vi "Write waveform to file.vi"(7 "File IO parameters":T1={"Output Folder"=path "C:/Users/Abigail/Documents/Imperial Optical software/Optical Software Code Simplified/Output", "Error file"=path "Error Log.txt", "Config file"=path "Config.ini", "File prefix"="", "Waveform read"={"t0"=timestamp(0 s since 1904-01-01), "dt"=1.0, "Y"=[]}}, 8 "error in":errorcluster, 10 "Dataset name":string="DAQ (raw data)", 11 "Data":dbl[][](array[numeric])) -> (0 "error out":errorcluster)   [LabVIEW 2017, in "File IO.lvlib"]
uses:
  File IO.lvlib
  Controls/Params.ctl
  <vilib>/Utility/file.llb/Write To Spreadsheet File (DBL).vi
panel:
  in  "Waveform":waveform(dbl)={"t0"=timestamp(3604668038.5453954 s since 1904-01-01), "dt"=1.0, "Y"=array[495 elements]}
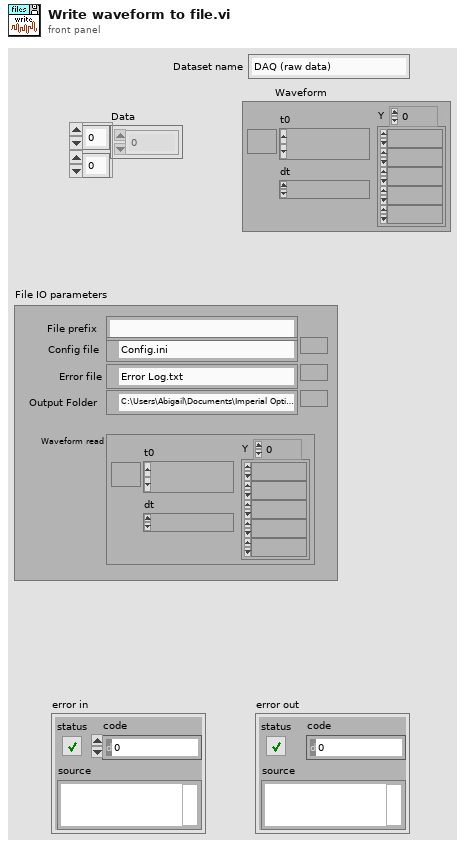
[diagram p1: front panel]
types:
  T1 = typedef "File IO.lvlib/Params.ctl" = cluster{"Output Folder":path, "Error file":path, "Config file":path, "File prefix":string, "Waveform read":waveform(dbl)}
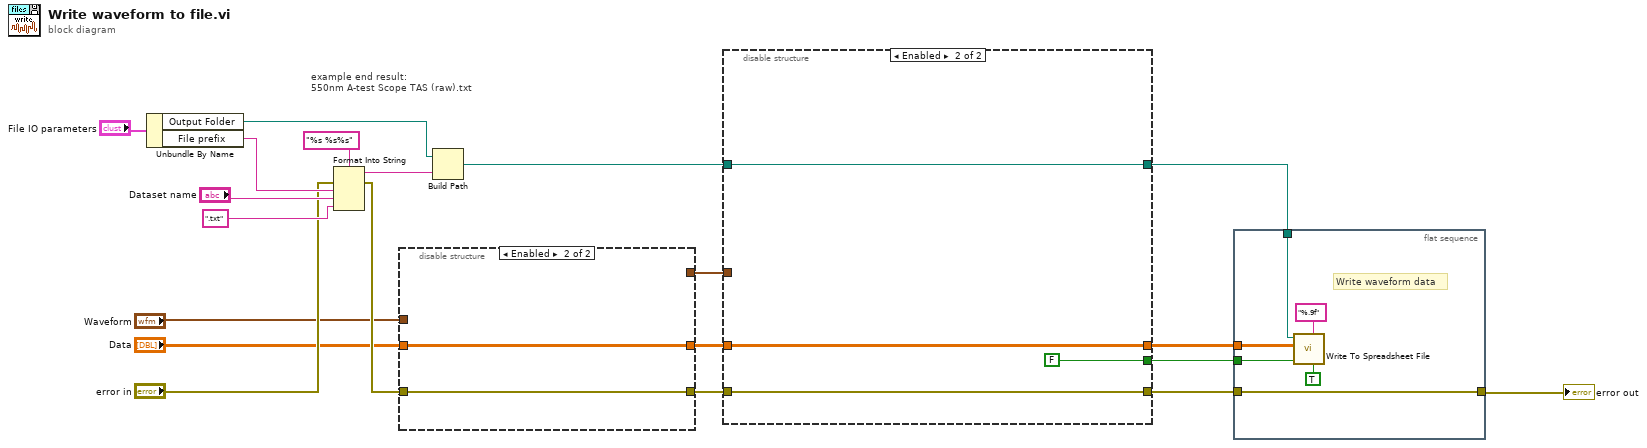
[diagram p0: block diagram]
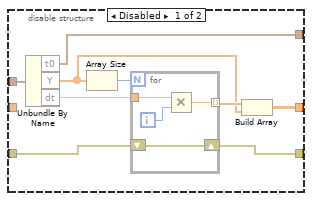
[diagram p2: hidden frame]
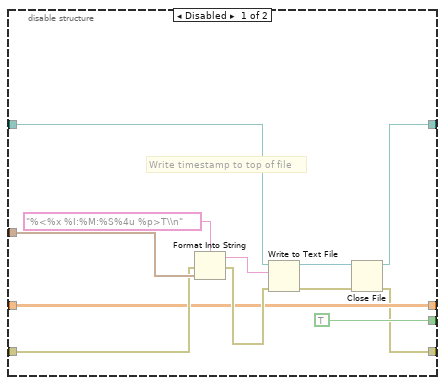
[diagram p3: hidden frame]
diagram:
  # "example end result:\n550nm A-test Scope TAS (raw).txt"
  n1 = Unbundle By Name("File IO parameters") -> ("Output Folder"=w20:path, "File prefix"=w19:string)
  n2 = Format Into String(format string="%s %s%s", error in="error in", w19, "Dataset name", ".txt" ("Dataset name 2")) -> (resulting string=w15:string, error out=w12:errorcluster)  [unwired: 1 in]
  n3 = disable-structure shown="Enabled" {
    disable-tunnel: w12 -> [w27 w34]
    disable-tunnel: "Waveform" -> [w24 _]
    disable-tunnel: [w23 _] -> w9
    disable-tunnel: [w22 w34] -> w8
    disable-tunnel: [w21 w35] -> w4
    disable-tunnel: "Data" -> [_ w35]
    frame Disabled {
      n4 = Unbundle By Name(w24) -> ("t0"=w23:timestamp, "Y"=w25:dbl[], "dt"=w28:dbl)
      n5 = Array Size(array=w25) -> (size(s)=w29:i32)
      n6 = for {
        N: w29 -> [_]
        tunnel: w28 -> [w33]
        shift-right: [w31] -> w22
        shift-left: w27 -> [w31]
        tunnel: [w30] -> w26 mode=indexing
        i -> [w32]
        n7 = Multiply(x=w33, y=w32) -> (x*y=w30:dbl)
      }
      n8 = Build Array(w26, w25) -> (w21:dbl[][])
    }
    frame Enabled {
    }
  }
  n9 = Build Path(base path=w20, name or relative path=w15) -> (appended path=w11:path)
  n10 = disable-structure shown="Enabled" {
    disable-tunnel: w11 -> [w39 w49]
    disable-tunnel: [w36 w51] -> w2
    disable-tunnel: w9 -> [w46 _]
    disable-tunnel: w8 -> [w45 w51]
    disable-tunnel: [TRUE ("append to file? (new file:F)") FALSE ("append to file? (new file:F)")] -> w5
    disable-tunnel: w4 -> [w41 w50]
    disable-tunnel: [w41 w50] -> w6
    disable-tunnel: [w38 w49] -> w7
    frame Disabled {
      # "Write timestamp to top of file"
      n11 = Format Into String(format string="%<%x %I:%M:%S%4u %p>T\\n" ("time format string (%c)"), error in=w45, w46) -> (resulting string=w43:string, error out=w44:errorcluster)  [unwired: 1 in]
      n12 = Write to Text File(file (use dialog)=w39, text=w43, error in=w44) -> (refnum out=w40:refnum<file>, error out=w37:errorcluster)  [unwired: 1 in, 1 out]
      n13 = Close File(refnum=w40, error in=w37) -> (path=w38:path, error out=w36:errorcluster)
    }
    frame Enabled {
    }
  }
  n14 = flat-sequence {
    tunnel: w7 -> [w57]
    tunnel: w6 -> [w56]
    tunnel: w5 -> [w55]
    tunnel: w2 -> [w52]
    tunnel: [w52] -> w1
    frame #0 {
      # "Write waveform data"
      n15 = call-poly <vilib>:"Write To Spreadsheet File.vi"("transpose? (no:F)"=TRUE, "format (%.3f)"="%.9f", "append to file? (new file:F)"=w55, "2D data"=w56, "file path (dialog if empty)"=w57) -> ()  [unwired: 3 in, 1 out]
    }
  }
  "error out" <- w1
